vi "Test Write.vi"() -> ()   [LabVIEW 2019, in "Control Experiment.lvclass"]
uses:
  Control Experiment.lvclass
panel:
  in  "stop":bool
  in  "Experiment Folder":string="6H_IVcurves"
  in  "Experiment Comments":string="SA03036H\nsweep Vsg:-150mV to 600mV, 1mV steps\nB: 7T to -7T\nVbg = -3.9V\nT: 50mK\n\nlockin\n\nI+/-: 2/3 3mV ac+ 250uV dc bias, 0.4 Hz\nV1+/-: 8/4\nV2+/- 6/28\nV3+/V3-: 27/8\nVsg: 1\nVbg :26\n\ntc 300ms order 2"
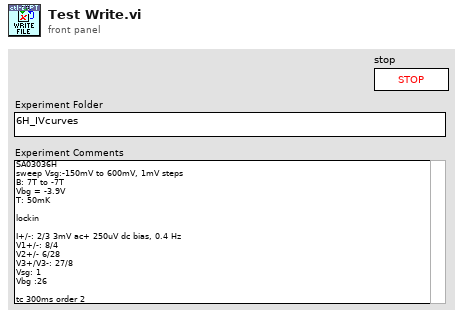
[diagram p1: front panel]
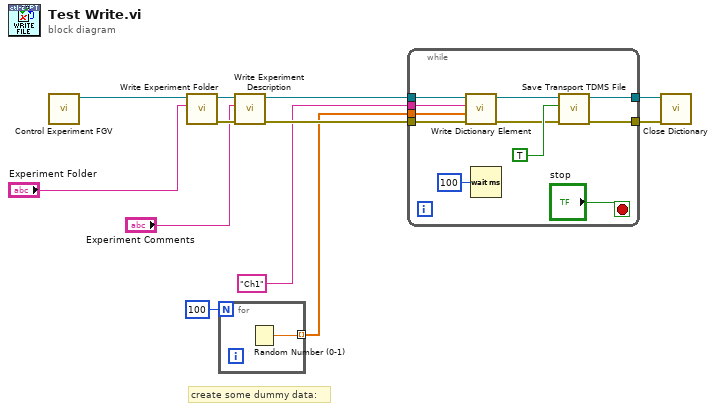
[diagram p0: block diagram]
diagram:
  # "create some dummy data:"
  n1 = call "Control Experiment FGV.vi"() -> ("Control Experiment.lvclass out"=w1:refnum<class "Control Experiment.lvclass">)  [unwired: 10 in, 1 out]
  n2 = call "Write Experiment Folder.vi"("Experiment Folder"="Experiment Folder", "Control Experiment in"=w1) -> ("error out"=w11:errorcluster, "Control Experiment out"=w12:refnum<class "Control Experiment.lvclass">)  [unwired: 8 in]
  n3 = for {
    N: 100 -> [_]
    tunnel: [w13] -> w4 mode=indexing
    n4 = Random Number (0-1)() -> (number: 0 to 1=w13:dbl)
  }
  n5 = call "Write Experiment Description.vi"("error in (no error)"=w11, "Experiment Description"="Experiment Comments", "Control Experiment in"=w12) -> ("error out"=w9:errorcluster, "Control Experiment out"=w8:refnum<class "Control Experiment.lvclass">)  [unwired: 7 in]
  n6 = while {
    tunnel: w9 -> [w21]
    tunnel: w8 -> [w20]
    tunnel: "Ch1" ("key") -> [w19]
    tunnel: w4 -> [w18]
    tunnel: [w16] -> w3
    tunnel: [w15] -> w2
    stop <- "stop" stop-if-true
    n7 = call "Write Dictionary Element.vi"("error in (no error)"=w21, "value"=w18, "key"=w19, "Control Experiment in"=w20) -> ("error out"=w22:errorcluster, "Control Experiment out"=w23:refnum<class "Control Experiment.lvclass">)  [unwired: 6 in]
    n8 = Wait (ms)(milliseconds to wait=u32 100) -> ()  [unwired: 1 out]
    n9 = call "Save Transport TDMS File.vi"("error in (no error)"=w22, "append?"=TRUE, "Control Experiment in"=w23) -> ("error out"=w16:errorcluster, "Control Experiment out"=w15:refnum<class "Control Experiment.lvclass">)  [unwired: 7 in]
  }
  n10 = call "Close Dictionary.vi"("error in (no error)"=w3, "Control Experiment in"=w2) -> ()  [unwired: 8 in, 2 out]
